vi "Handshake_PostUUT.vi"(8 "error in":errorcluster, 9 "Tester Tx":T2={"Fault"=FALSE, "StepNo"=0, "Ready"=TRUE, "HighVoltage"=FALSE, "TestRunning"=FALSE, "ResultsReady"=FALSE, "Results"=0, "ElapsedTime"=0, "Online"=TRUE, "TimeCompleted"=[], "Timeout"=FALSE}, 10 "Tester Rx In":T1={"Start"=FALSE, "NestStatus"=FALSE, "PalletID"=0, "BarcodeData"="P:10-000001R:04S:QMC2200001", "StepEcho"=0, "Cylinder_1"=FALSE, "Cylinder_2"=FALSE, "Cylinder_3"=FALSE, "Cylinder_4"=FALSE, "Cylinder_5"=FALSE, "ResultsAck"=FALSE, "Reset"=FALSE, "Stop"=FALSE, "FaultCode"=0}) -> (0 "error out":errorcluster, 2 "Tester Rx out":T1)   [LabVIEW 2021, in "Panel.lvlib" / "Panel.lvclass"]
uses:
  Panel.lvclass
  Type Defs/Tester Rx Dataset.ctl
  Type Defs/Tester Tx Dataset.ctl
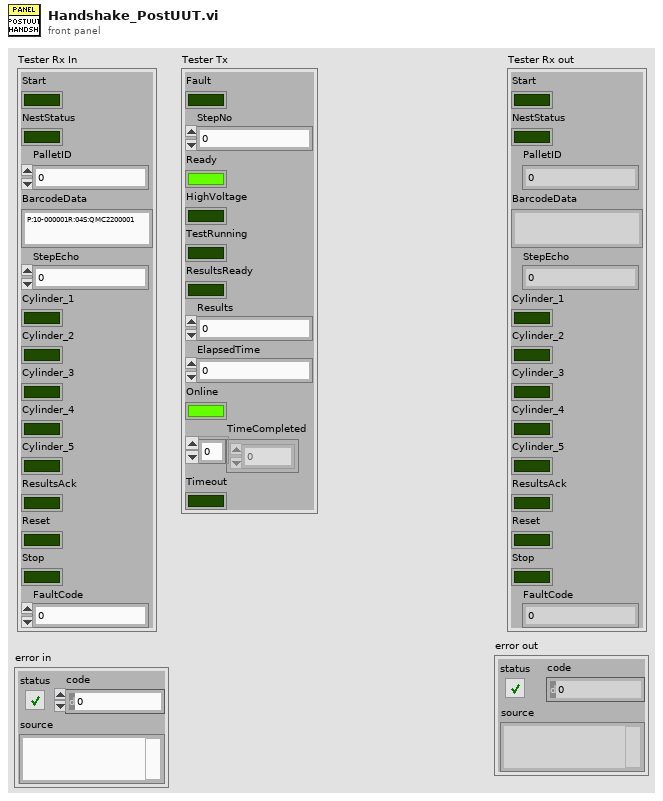
[diagram p1: front panel]
types:
  T1 = typedef "Panel.lvlib/Panel.lvclass/Tester Rx Dataset.ctl" = cluster{"Start":bool, "NestStatus":bool, "PalletID":u32, "BarcodeData":string, "StepEcho":u32, "Cylinder_1":bool, "Cylinder_2":bool, "Cylinder_3":bool, "Cylinder_4":bool, "Cylinder_5":bool, "ResultsAck":bool, "Reset":bool, "Stop":bool, "FaultCode":u32}
  T2 = typedef "Panel.lvlib/Panel.lvclass/Tester Tx Dataset.ctl" = cluster{"Fault":bool, "StepNo":u32, "Ready":bool, "HighVoltage":bool, "TestRunning":bool, "ResultsReady":bool, "Results":u32, "ElapsedTime":u32, "Online":bool, "TimeCompleted":i32[], "Timeout":bool}
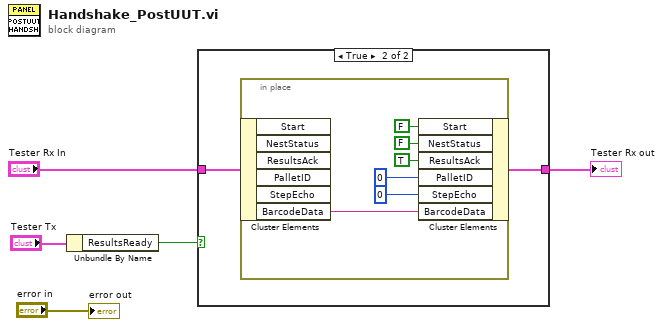
[diagram p0: block diagram]
diagram:
  n1 = Unbundle By Name("Tester Tx") -> ("ResultsReady"=w4:bool)
  n2 = case shown="True" w4 {
    tunnel: "Tester Rx In" -> [w6 w8]
    tunnel: [w6 w7] -> w1
    frame False {
    }
    frame True {
      n3 = in-place {
        n4 = in-place-cluster #1(w8) -> ("BarcodeData"=w12:string)  [unwired: 5 out]
        n5 = in-place-cluster #1("Start"=FALSE, "NestStatus"=FALSE, "ResultsAck"=TRUE, "PalletID"=u32 0, "StepEcho"=u32 0, "BarcodeData"=w12) -> (w7:T1)
      }
    }
  }
  "Tester Rx out" <- w1
  "error out" <- "error in"
